vi "Test Exisitng Recieved File is Deleted if Test Passes.vi"(11 "Test Case In":refnum<class "Basic Mechanics Tests.lvclass">) -> (0 "error out":errorcluster, 3 "Test Case Out":refnum<class "Basic Mechanics Tests.lvclass">)   [LabVIEW 2020, in "Basic Mechanics Tests.lvclass"]
uses:
  Basic Mechanics Tests.lvclass
  Basic Mechanics Tests.lvclass/Basic Mechanics Tests.ctl
  C:/Program Files/National Instruments/LabVIEW 2025/vi.lib/Astemes/LUnit/Test Case.lvclass
  C:/Program Files/National Instruments/LabVIEW 2025/vi.lib/Astemes/LUnit/LUnit Runnable.lvclass
  C:/Users/SAS/Desktop/ApprovalTests.LabVIEW/Tests/Basic Mechanics Tests/Basic Mechanics Tests.lvclass
  Source/Approval Tests/Report Nothing/Report Nothing.lvclass
  C:/Users/SAS/Desktop/ApprovalTests.LabVIEW/Source/Approval Tests/Report Nothing/Report Nothing.lvclass
  C:/Users/SAS/Desktop/ApprovalTests.LabVIEW/Source/Approval Tests/Reporter/Reporter.lvclass
  4be351cf-9afa-44a9-9686-c31d6937e1da.vi
  Source/Approval Tests/Options/Options.lvclass
  <vilib>/Astemes/LUnit/Test Case.lvclass
  fbf3a6f1-25d3-4b1a-9ed1-fe282719be7b.vi
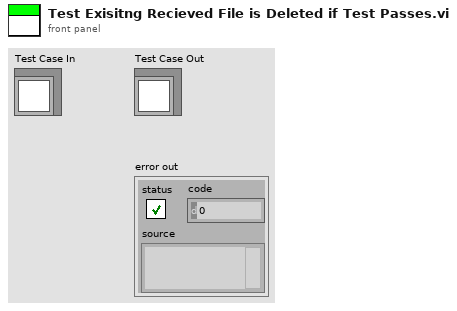
[diagram p1: front panel]
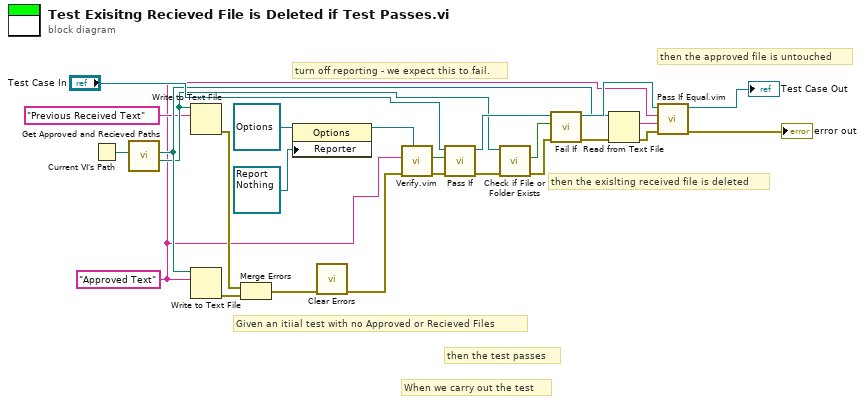
[diagram p0: block diagram]
diagram:
  w1 = "Approved Text"
  # "then the approved file is untouched"
  # "then the exislting received file is deleted"
  # "then the test passes"
  # "When we carry out the test"
  # "Given an itiial test with no Approved or Recieved Files"
  # "turn off reporting - we expect this to fail."
  n1 = Current VI's Path() -> (path=w10:path)
  n2 = call "Get Approved and Recieved Paths.vi"("This VI"=w10) -> ("Recieved"=w4:path, "Approved Path"=w6:path)  [unwired: 9 in]
  n3 = Write to Text File(file (use dialog)=w4, text="Previous Received Text") -> (error out=w2:errorcluster)  [unwired: 2 in, 2 out]
  n4 = Write to Text File(file (use dialog)=w6, text=w1) -> (error out=w5:errorcluster)  [unwired: 2 in, 2 out]
  n5 = Merge Errors(w2, w5) -> (w21:errorcluster)
  n6 = property on="Property Node" class="Options"(reference=refnum<class "Options.lvclass"> refnum ("Options"), "Reporter"=refnum<class "Report Nothing.lvclass"> refnum ("Approval Tests.lvlib:Report Nothing")) -> (reference out=w17:refnum<class "Options.lvclass">)  [unwired: 1 in, 1 out]
  n7 = call <vilib>:"Clear Errors.vi"("error in (no error)"=w21) -> ("error out"=w20:errorcluster)  [unwired: 5 in, 1 out]
  n8 = call "Verify.vim"("Options"=w17, "error in"=w20, "Anything"=w1) -> ("error out"=w22:errorcluster, "Passed?"=w15:bool)  [unwired: 6 in, 1 out]
  n9 = call <vilib>:"Pass If.vi"("error in (no error)"=w22, "Pass?"=w15, "LUnit Test Case In"="Test Case In") -> ("error out"=w9:errorcluster, "LUnit Test Case Out"=w14:refnum<class "Basic Mechanics Tests.lvclass">)  [unwired: 7 in]
  n10 = call <vilib>:"Check if File or Folder Exists.vi"("error in (no error)"=w9, "path"=w4) -> ("error out"=w8:errorcluster, "file or folder exists?"=w7:bool)  [unwired: 7 in, 1 out]
  n11 = call <vilib>:"Fail If.vi"("error in (no error)"=w8, "Fail?"=w7, "LUnit Test Case In"=w14) -> ("error out"=w23:errorcluster, "LUnit Test Case Out"=w13:refnum<class "Basic Mechanics Tests.lvclass">)  [unwired: 7 in]
  n12 = Read from Text File(file (use dialog)=w6, error in=w23) -> (text=w11:string, error out=w24:errorcluster)  [unwired: 2 in, 2 out]
  n13 = call "Pass If Equal.vim"("error in (no error)"=w24, "Actual"=w11, "Expected"=w1, "LUnit Test Case In"=w13) -> ("error out"=→"error out":errorcluster, "LUnit Test Case Out"=→"Test Case Out":refnum<class "Basic Mechanics Tests.lvclass">)  [unwired: 6 in]
